vi "Auto-Cycle.vi"(8 "error in (no error)":errorcluster, 11 "SJ-210 in":refnum<class "SJ-210.lvclass">) -> (0 "error out":errorcluster, 3 "SJ-210 out":refnum<class "SJ-210.lvclass">)   [LabVIEW 2014, in "SJ-210.lvlib" / "SJ-210.lvclass"]
doc: "Auto ciclo encargado de iniciar la adquisición de datos, esperar hasta que finalice el proceso y lee el buffer para extraer los valores que luego serán enviados al cluster de datos."
uses:
  SJ-210.lvclass
  SJ-210.lvclass/SJ-210.ctl
  API/SJ-210 Lib.lvlib
  DriverMasterAsync/builds/DriverMasterAsync.lvlibp/Modules/HAL/DriverMasterAsync/DriverMasterAsyncClass/DriverMasterAsync.lvclass
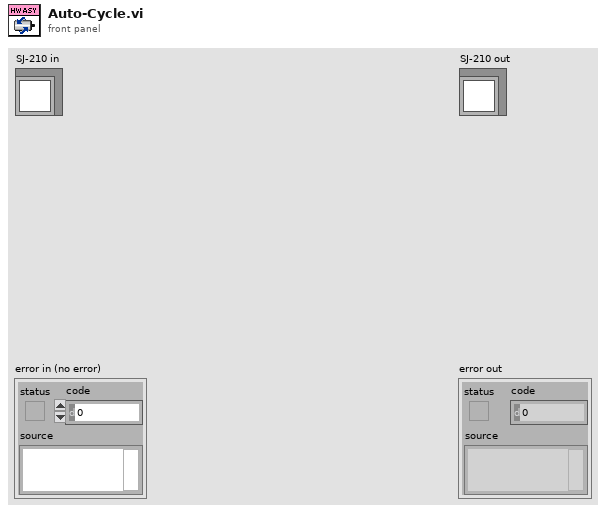
[diagram p1: front panel]
types:
  T1 = cluster{"VISA resource name":refnum<visa-resource-name>}
  T2 = typedef "SJ-210 Lib.lvlib/Connection Data.ctl" = cluster{"VISA resource name":refnum<visa-resource-name>}
  T3 = typedef "SJ-210 Lib.lvlib/ACQ Data.ctl" = sgl[]
  T4 = typedef "DriverMasterAsync.lvlibp/WINFAS 2 Data Queue.lvlib/Async Acquisition Data Cluster.ctl" = cluster{"Data":sgl[]}
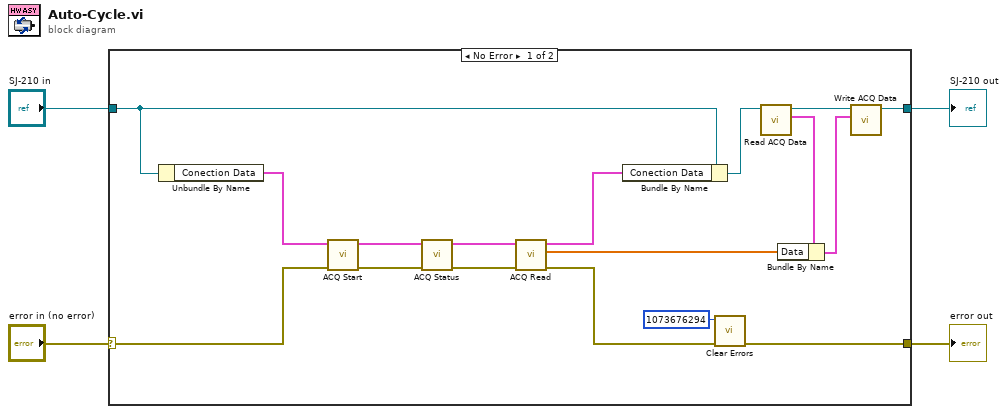
[diagram p0: block diagram]
diagram:
  n1 = case shown="No Error" "error in (no error)" {
    selector: "error in (no error)" -> [w11 w23]
    tunnel: [w5 w23] -> w3
    tunnel: [w14 w22] -> w1
    tunnel: "SJ-210 in" -> [w9 w22]
    frame No Error {
      n2 = Unbundle By Name(w9) -> ("Conection Data"=w12:T1)
      n3 = call "ACQ Start.vi"("error in (no error)"=w11, "Conection Data"=w12) -> ("error out"=w19:errorcluster, "Conection Data Out"=w21:T2)  [unwired: 8 in]
      n4 = call "ACQ Status.vi"("error in (no error)"=w19, "Conection Data"=w21) -> ("error out"=w18:errorcluster, "Conection Data Out"=w20:T2)  [unwired: 8 in]
      n5 = call "ACQ Read.vi"("error in (no error)"=w18, "Conection Data"=w20) -> ("error out"=w6:errorcluster, "ACQ Data"=w16:T3, "Conection Data Out"=w10:T2)  [unwired: 7 in]
      n6 = Bundle By Name(cluster=w9, "Conection Data"=w10) -> (w8:refnum<class "SJ-210.lvclass">)
      n7 = call <vilib>:"Clear Errors.vi"("error in (no error)"=w6, "specific error code to clear (0: all)"=1073676294) -> ("error out"=w5:errorcluster)  [unwired: 4 in, 1 out]
      n8 = call "Read ACQ Data.vi"("DriverMasterAsync in"=w8) -> ("ACQ Data"=w17:T4, "DriverMasterAsync out"=w13:refnum<class "SJ-210.lvclass">)  [unwired: 8 in, 1 out]
      n9 = Bundle By Name(cluster=w17, "Data"=w16) -> (w15:T4)
      n10 = call "Write ACQ Data.vi"("ACQ Data"=w15, "DriverMasterAsync in"=w13) -> ("DriverMasterAsync out"=w14:refnum<class "SJ-210.lvclass">)  [unwired: 8 in, 1 out]
    }
    frame Error {
    }
  }
  "error out" <- w3
  "SJ-210 out" <- w1
